vi "BNC555.get i attribute.vi"(0 "i ref in":refnum<vi>, 5 "error in (no error)":errorcluster) -> (14 "i ref out":refnum<vi>, 16 "i attribute":T1={"Information"={"VISA resource name"="", "Baud Rate (1:9600)"=1}, "Channel Array"=[], "System"={"Sys Period"=0.0, "Sys Oscillator"=FALSE, "Sys Mode"=enum."Normal", "Sys Burst #"=0, "Sys DC On"=10, "Sys DC Off"=5, "Sys Trig Mode"=enum."Gated", "Sys Trig Lev"=2.5, "Sys Gate State"=TRUE, "Sys Trig Edge"=TRUE, "Sys State"=TRUE}, "GUI Refs"={"Delete"=refnum, "Information"=refnum, "System"=refnum, "Channel Array"=refnum, "Device Error"=refnum, "Instr Driver Revision"=refnum, "Instr Firmware Revision"=refnum, "Instr Option"=refnum, "Self-Test Response"=refnum}, "Service IDs Channelinfo"=[-1], "Service ID T0 Mode"=-1} {"System"."Sys Period" format="%.6p"; "System"."Sys Trig Lev" format="%.4p"; "Channel Array"."Chan Lev Adjust" format="%.3p"; "Channel Array"."Chan Width" format="%.3p"; "Channel Array"."Chan Delay" format="%.3p"; "Channel Array"."Chan #" items=["System (To)", "Channel A", "Channel B", "Channel C", "Channel D", "Channel E", "Channel F", "Channel G", "Channel H"]; "Information"."Baud Rate (1:9600)" items=["4800", "9600", "19200", "38400"]}, 19 "error out":errorcluster)   [LabVIEW 2014, in "BNC555.lvlib"]
doc: "Gets the i attribute data of an object.\n\nLicense Agreement for this software:\n\nCopyright (C)\nGesellschaft für Schwerionenforschung, GSI\nPlanckstr. 1\n64291 Darmstadt\nGermany\n\nContact: D.Beck@gsi.de \n\nThis program is free software; you can redistribute it and/or modify it under the terms of the GNU General Public License as published by the Free Software Foundation; either version 2 of the license, or (at your option) any later version.\n\nThis program is distributed in the hope that it will be useful, but WITHOUT ANY WARRANTY; without even the implied warranty of MERCHANTABILITY or FITNESS FOR A PARTICULAR PURPOSE. See the GNU General License for more details (http://www.gnu.org).\n\nGesellschaft für Schwerionenforschung, GSI\nPlanckstr. 1, 64291 Darmstadt, Germany\nFor all questions and ideas contact: M.Richter@gsi.de, H.Brand@gsi.de or D.Beck@gsi.de.\nLast update: 17-JUN-2004"
uses:
  BNC555.lvlib
  BNC555.i attribute.ctl
  non_GPL/instr.lib/BNC555/BNC555_U.llb/BNC555 All Chan Parameters.ctl
  non_GPL/instr.lib/BNC555/BNC555_U.llb/BNC555 All Sys Parameters.ctl
  non_GPL/instr.lib/BNC555/BNC555 - Driver np.lvlib
panel:
  # "Run\nStop"
  # "System (To) Mode"
  # "Triggering"
  # "High\nLow"
  # "Rising\nFalling"
  # "External\nInternal"
  # "Output"
  # "Gate"
  # "On\nOff"
  # "Pulse"
  # "On\nOff"
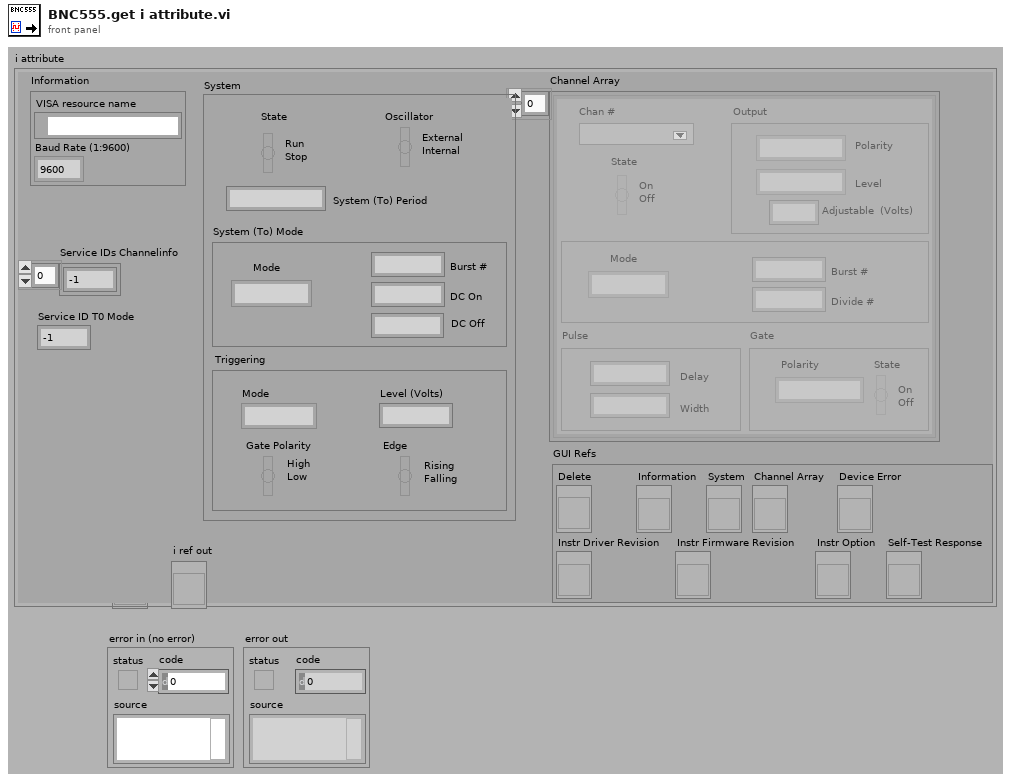
[diagram p1: front panel]
types:
  T1 = typedef "BNC555.lvlib/BNC555.i attribute.ctl" = cluster{"Information":cluster{"VISA resource name":refnum<visa-resource-name>, "Baud Rate (1:9600)":u16}, "Channel Array":T2[], "System":T3, "GUI Refs":cluster{"Delete":refnum<vi>, "Information":refnum<vi>, "System":refnum<vi>, "Channel Array":refnum<vi>, "Device Error":refnum<vi>, "Instr Driver Revision":refnum<vi>, "Instr Firmware Revision":refnum<vi>, "Instr Option":refnum<vi>, "Self-Test Response":refnum<vi>}, "Service IDs Channelinfo":i32[], "Service ID T0 Mode":i32}
  T2 = typedef "BNC555 - Driver np.lvlib/BNC555 All Chan Parameters.ctl" = cluster{"Chan #":i32, "Chan State":bool, "Chan Delay":dbl, "Chan Width":dbl, "Chan Mode":enum16{"Normal", "Single", "Burst", "Divide by N"}, "Chan Burst #":u32, "Chan Divide #":u32, "Chan Pol Out":enum16{"Normal", "Complement", "Inverted"}, "Chan Level Out":enum16{"TTL", "Adjustable", "35 Volt"}, "Chan Lev Adjust":dbl, "Chan Gate Pol":enum16{"Normal", "Complement", "Inverted"}, "Chan Gate State":bool}
  T3 = typedef "BNC555 - Driver np.lvlib/BNC555 All Sys Parameters.ctl" = cluster{"Sys Period":dbl, "Sys Oscillator":bool, "Sys Mode":enum16{"Normal", "Single", "Burst", "Duty Cycle"}, "Sys Burst #":u32, "Sys DC On":u32, "Sys DC Off":u32, "Sys Trig Mode":enum16{"Disabled", "Triggered", "Gated"}, "Sys Trig Lev":dbl, "Sys Gate State":bool, "Sys Trig Edge":bool, "Sys State":bool}
  T4 = enum16{"SetAttribute", "GetAttribute", "CreateAttribute", "DestroyAttribute", "DestroyAllAtributes"}
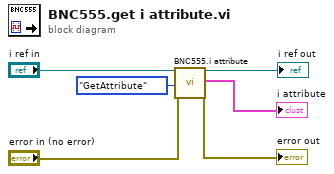
[diagram p0: block diagram]
diagram:
  n1 = call "BNC555.i attribute.vi"("VI Refnum"="i ref in", "Action"=T4."GetAttribute", "error in (no error)"="error in (no error)") -> ("VI Refnum out"=→"i ref out":refnum<vi>, "CLASS.i attribute out"=→"i attribute":T1, "error out"=→"error out":errorcluster)  [unwired: 14 in]
